vi "slscsl_connect.vi"(8 "error in (no error)":errorcluster, 10 "connectionList":string, 11 "slscsl in":refnum<class "slscsl.lvclass">) -> (0 "error out":errorcluster, 2 "switchActionsArray":T1 {"RelayAction" items=["CloseRelay"=21, "OpenRelay"=20]}, 3 "slscsl out":refnum<class "slscsl.lvclass">)   [LabVIEW 2015, in "SLSC Switch.lvlib" / "slscsl.lvclass"]
uses:
  slscsl.lvclass
  RelayAction.ctl
  SwitchAction.ctl
  SwitchActionsArray.ctl
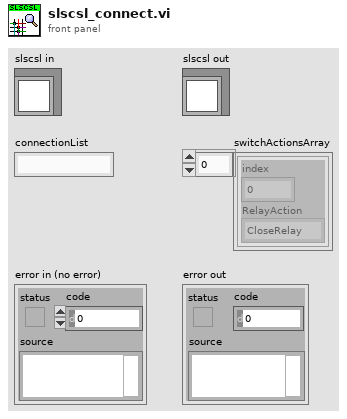
[diagram p1: front panel]
types:
  T1 = typedef "SLSC Switch.lvlib/slscsl.lvclass/SwitchActionsArray.ctl" = T2[]
  T2 = typedef "SLSC Switch.lvlib/slscsl.lvclass/SwitchAction.ctl" = cluster{"index":i32, "RelayAction":T3}
  T3 = typedef "SLSC Switch.lvlib/slscsl.lvclass/RelayAction.ctl" = u32
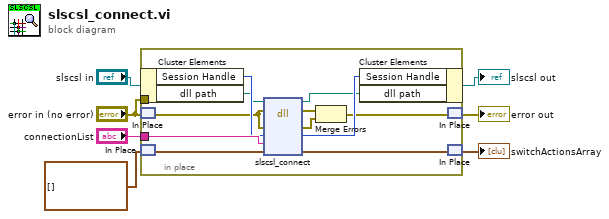
[diagram p0: block diagram]
diagram:
  n1 = in-place {
    in-place-border: "error in (no error)" -> [_]
    in-place-border: "connectionList" -> [w15]
    n2 = in-place-cluster #1("slscsl in") -> ("Session Handle"=w14:u64, "dll path"=w9:path)
    n3 = in-place-match #2("error in (no error)") -> (w13:errorcluster)
    n4 = in-place-match #3(T1 [] ("SwitchActionList")) -> (w11:T1)
    n5 = dll-call lib="?" fn="slscsl_connect"(path in=w9, error in=w13, "errorCluster"=w13, "sessionHandle"=w14, "connectionList"=w15, "switchActionsArray"=w11) -> (path out=w8:path, error out=w18:errorcluster, "errorCluster"=w17:errorcluster, "sessionHandle"=w16:u64, "switchActionsArray"=w10:T1)  [unwired: 3 in]
    n6 = Merge Errors(w18, w17) -> (w12:errorcluster)
    n7 = in-place-cluster #1("Session Handle"=w16, "dll path"=w8) -> (→"slscsl out":refnum<class "slscsl.lvclass">)
    n8 = in-place-match #2(w12) -> (→"error out":errorcluster)
    n9 = in-place-match #3(w10) -> (→"switchActionsArray":T1)
  }
